vi "New Entity UI.vi"(10 "Target Name":string, 11 "Project Name":string) -> (2 "Cancelled":bool, 3 "Entity Name":string)   [LabVIEW 2020, in "Conditum-Tools.lvlib" / "Entity Editor.lvclass"]
uses:
  Entity Editor.lvclass
  Entity Editor.lvclass/Entity Editor.ctl
panel:
  out "Message":string
  in  "Cancel":bool
  in  "OK":bool
  in  "Name":string
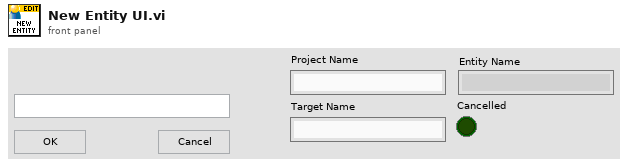
[diagram p1: front panel]
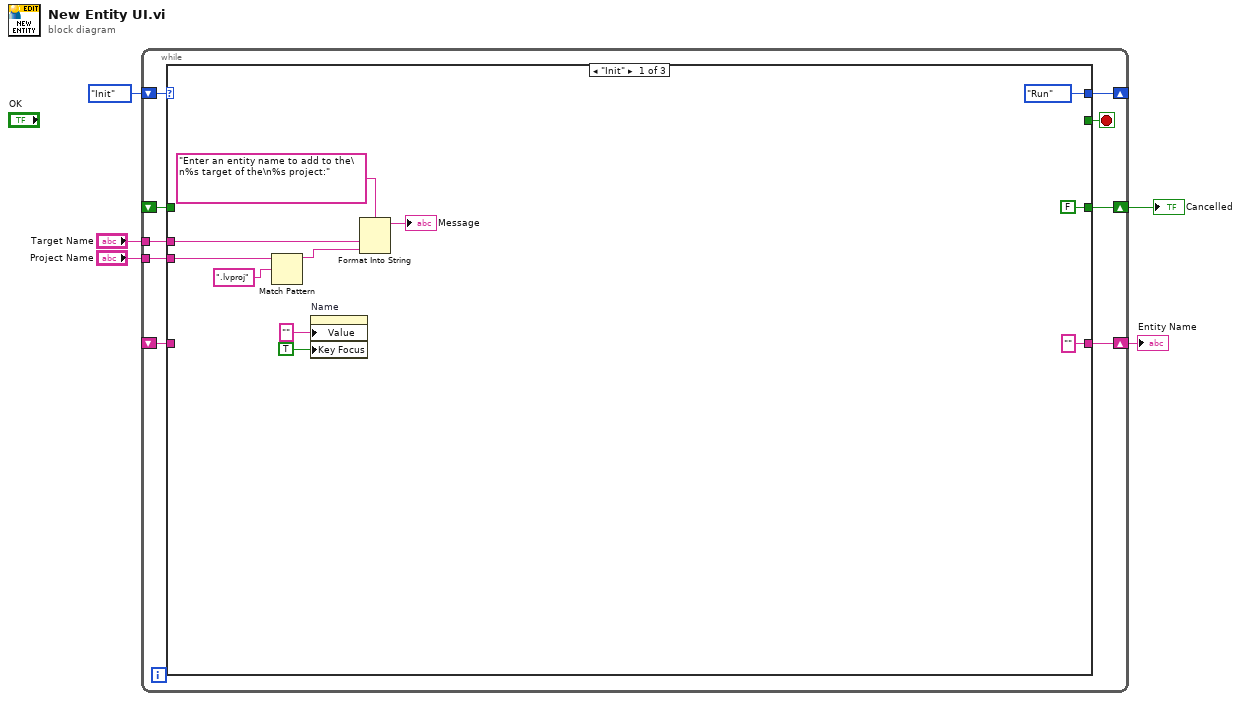
[diagram p0: block diagram]
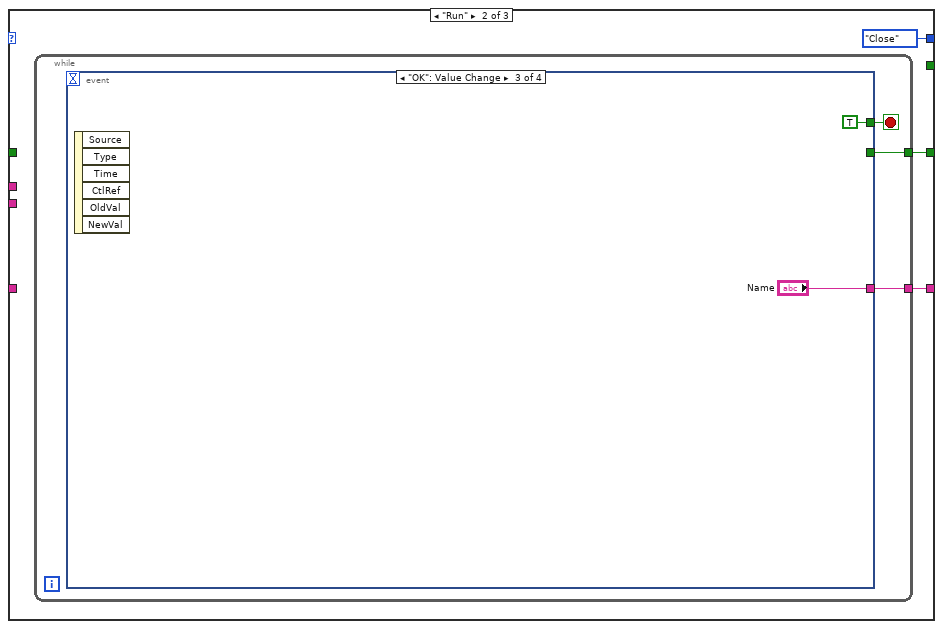
[diagram p2: hidden frame]
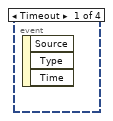
[diagram p3: hidden frame]
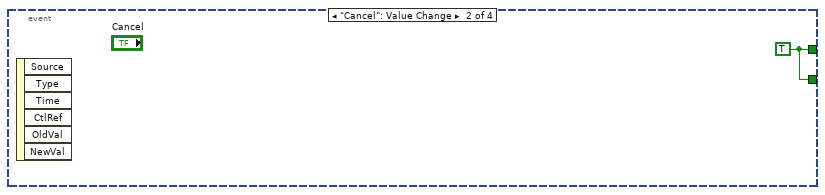
[diagram p4: hidden frame]
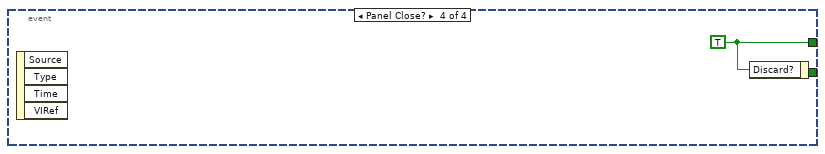
[diagram p5: hidden frame]
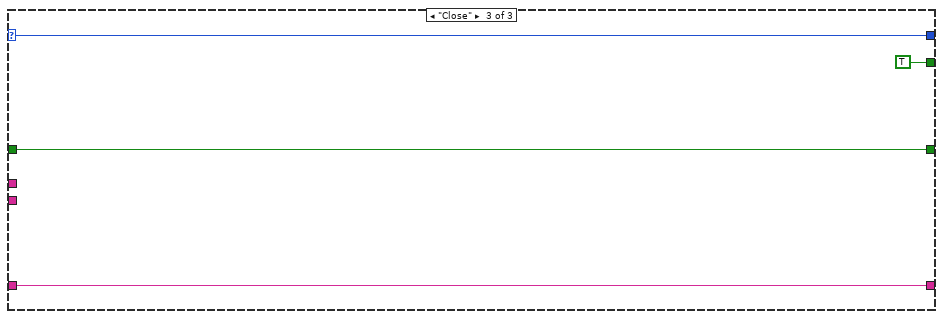
[diagram p6: hidden frame]
diagram:
  n1 = while {
    shift-right: [w13] -> _
    shift-left: enum16{"Init", "Run", "Close"}."Init" ("Basic UI State") -> [w14]
    tunnel: "Project Name" -> [w11]
    shift-right: [w10] -> w3
    shift-left: _ -> [w9]
    tunnel: "Target Name" -> [w8]
    shift-right: [w7] -> w1
    shift-left: _ -> [w6]
    stop <- w12 stop-if-true
    n2 = case shown="\"Init\"" w14 {
      selector: w14 -> [_ _ w39]
      tunnel: [enum16{"Init", "Run", "Close"}."Run" ("Basic UI State") enum16{"Init", "Run", "Close"}."Close" ("Basic UI State") w39] -> w13
      tunnel: [_ _ TRUE] -> w12
      tunnel: w11 -> [w20 _ _]
      tunnel: [FALSE w27 w37] -> w10
      tunnel: w9 -> [_ _ w37]
      tunnel: w8 -> [w22 _ _]
      tunnel: ["" ("Name") w26 w36] -> w7
      tunnel: w6 -> [_ _ w36]
      frame "Init" {
        n3 = Match Pattern(string=w20, regular expression=".lvproj") -> (before substring=w19:string)  [unwired: 1 in, 3 out]
        n4 = property on="Name" class="Str"("Value"="" ("Name"), "Key Focus"=TRUE) -> ()  [unwired: 2 in, 2 out]
        n5 = Format Into String(format string="Enter an entity name to add to the\n%s target of the\n%s project:" ("Message"), w22, w19) -> (resulting string=→"Message":string)  [unwired: 2 in, 1 out]
      }
      frame "Run" {
        n6 = while {
          tunnel: [w30] -> w27
          tunnel: [w29] -> w26
          stop <- w31 stop-if-true
          n7 = event shown="[2] \"OK\": Value Change" {
            selector: _ -> [_ _ _ _]
            dyn-events: _ -> [_ _ _ _]
            timeout: _ -> [_ _ _ _]
            tunnel: [_ w32 TRUE w35] -> w31
            tunnel: [_ w32 _ _] -> w30
            tunnel: [_ _ "Name" _] -> w29
            event Timeout {
              n8 = event-data() -> ()  [unwired: 1 in, 3 out]
            }
            event "Cancel": Value Change {
              w32 = TRUE
              n9 = event-data() -> ()  [unwired: 1 in, 6 out]
            }
            event "OK": Value Change {
              n10 = event-data() -> ()  [unwired: 1 in, 6 out]
            }
            event Panel Close? {
              w35 = TRUE
              n11 = event-data() -> ()  [unwired: 1 in, 4 out]
              n12 = event-data("Discard?"=w35) -> ()  [unwired: 1 in, 1 out]
            }
          }
        }
      }
      frame "Close" {
      }
    }
  }
  "Cancelled" <- w3
  "Entity Name" <- w1
